vi "Configure Value Hold.vi"(8 "error in (no error)":errorcluster, 9 "Measurement Number (0: <0>)":i32(ring) items=["Measurement 1"=1, "Measurement 2"=2, "Measurement 3"=3, "Measurement 4"=4], 10 "Hold State (0: OFF)":i32(ring) items=["OFF", "MIN", "MAX"], 11 "VISA resource name":refnum<visa-resource-name>) -> (0 "error out":errorcluster, 3 "VISA resource name out":refnum<visa-resource-name>)   [LabVIEW 2011, in "Agilent N432A.lvlib"]
doc: "Sets the minimum or maximum hold value of the power measured for the specified measurement."
uses:
  <instrlib>/Agilent N432A/Agilent N432A.lvlib
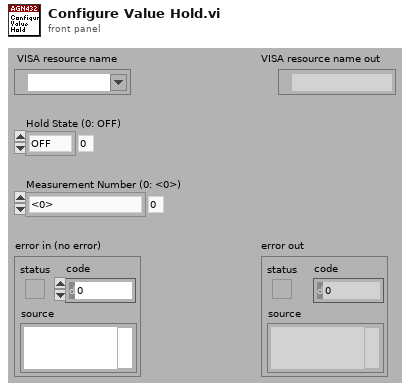
[diagram p1: front panel]
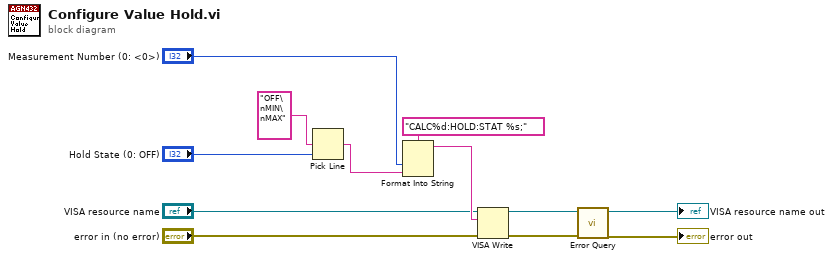
[diagram p0: block diagram]
diagram:
  n1 = Pick Line(multi-line string="OFF\nMIN\nMAX", line index="Hold State (0: OFF)") -> (output string=w8:string)  [unwired: 1 in]
  n2 = Format Into String(format string="CALC%d:HOLD:STAT %s;", "Measurement Number (0: <0>)", w8) -> (resulting string=w7:string)  [unwired: 2 in, 1 out]
  n3 = VISA Write(VISA resource name="VISA resource name", write buffer=w7, error in (no error)="error in (no error)") -> (VISA resource name out=w4:refnum<visa-resource-name>, error out=w3:errorcluster)  [unwired: 1 out]
  n4 = call <instrlib>:"Error Query.vi"("error in (no error)"=w3, "VISA resource name"=w4) -> ("error out"=→"error out":errorcluster, "VISA resource name out"=→"VISA resource name out":refnum<visa-resource-name>)  [unwired: 6 in, 2 out]
